vi "Modbus Initialization VI.vi"(8 "error in (no error)":errorcluster, 10 "Custom XML":string, 11 "Device Item Ref in":T1 format="%.0x") -> (0 "error out":errorcluster, 3 "Device Item Ref out":T1 format="%.0x")   [LabVIEW 2014, in "Modbus System Explorer.lvlib"]
uses:
  Modbus System Explorer.lvlib
  <vilib>/NI Veristand/Custom Device API/Custom Device Item Ref.ctl
  <vilib>/NI Veristand/Custom Device API/Custom Device Channel.ctl
  <vilib>/NI Veristand/Custom Device API/Custom Device Channel Type.ctl
  Glyphs/Modbus Property Names.vi
  Shared/Modbus GUID Lookup.vi
  <vilib>/NI Veristand/Custom Device API/Set Item Property (String).vi
  <vilib>/NI Veristand/Custom Device API/Set Item Property (Path).vi
  <vilib>/NI Veristand/Custom Device API/Custom Device API.lvlib
  Shared/Modbus Shared.lvlib
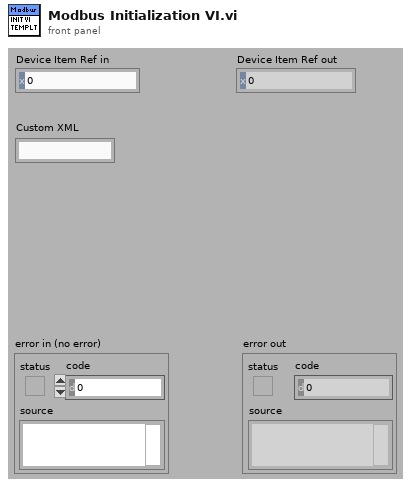
[diagram p1: front panel]
types:
  T1 = typedef "Custom Device API.lvlib/Custom Device Item Ref.ctl" = u64
  T2 = typedef "Custom Device API.lvlib/Custom Device Channel.ctl" = cluster{"Type":T3, "Units":string, "Default Value":dbl, "Faultable":bool, "Scalable":bool}
  T3 = typedef "Custom Device API.lvlib/Custom Device Channel Type.ctl" = enum16{"Input", "Output"}
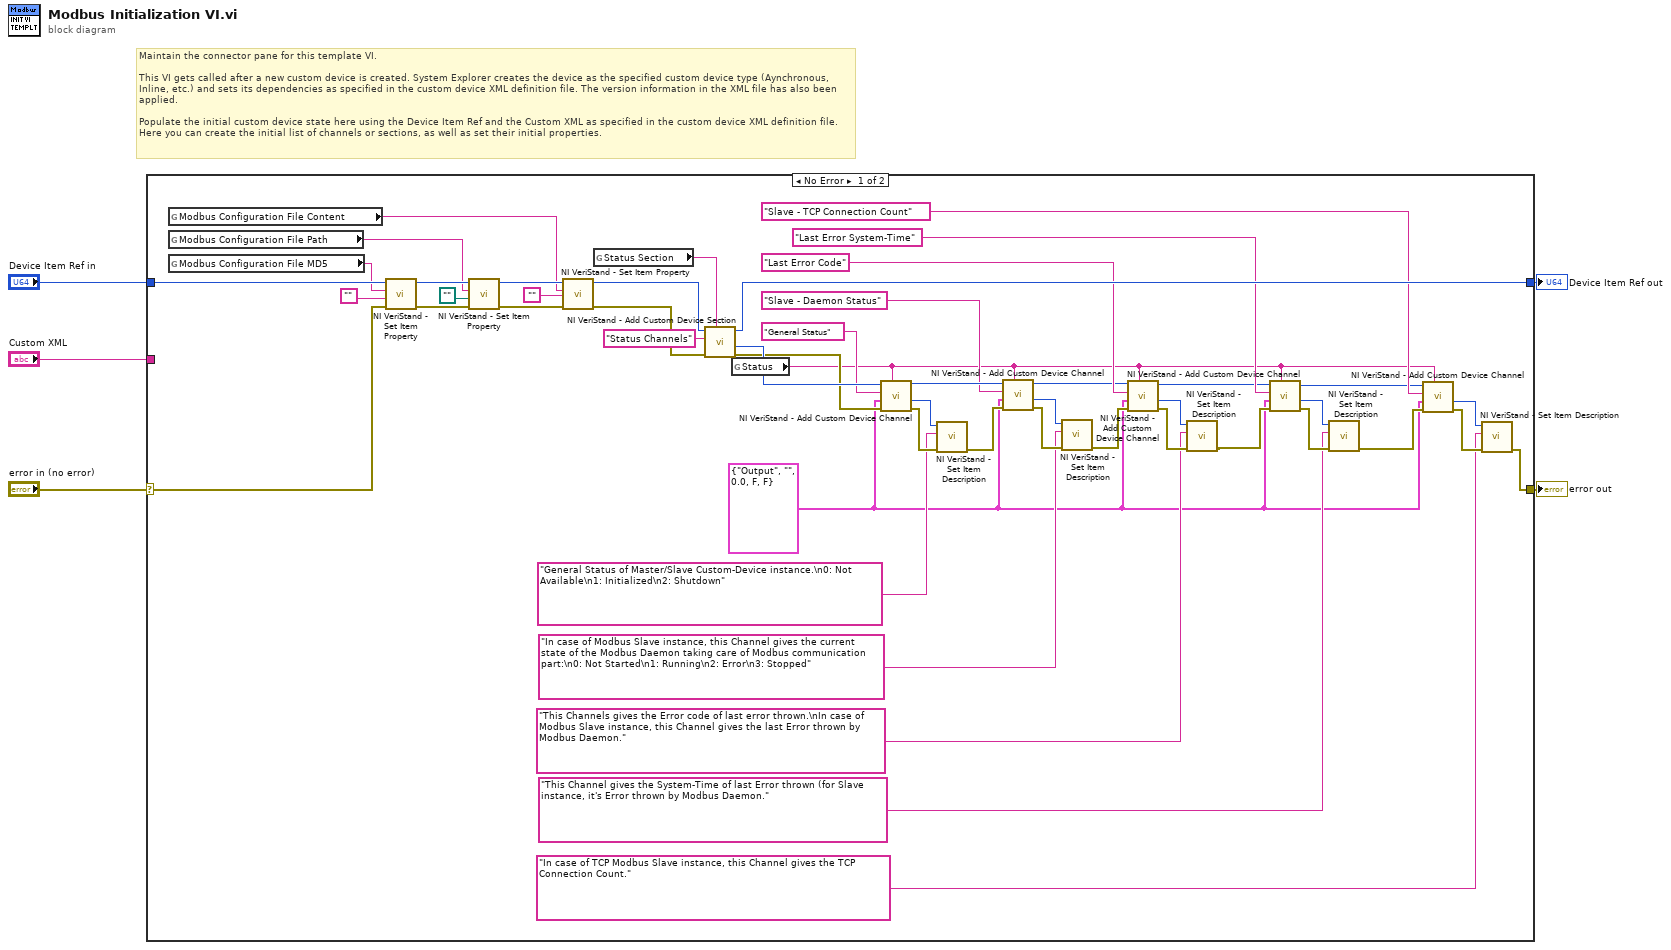
[diagram p0: block diagram]
diagram:
  # "Maintain the connector pane for this template VI.\n\nThis VI gets called after a new custom device is created. System Explorer creates the device as the specified custom device type (Aynchronous, Inline, etc.) and sets its dependencies as specified in the custom device XML definition file. The version information in the XML file has also been applied.\n\nPopulate the initial custom device state here using the Device Item Ref and the Custom XML as specified in the custom device XML definition file. Here you can create the initial list of channels or sections, as well as set their initial properties."
  n1 = case shown="No Error" "error in (no error)" {
    selector: "error in (no error)" -> [w52 w57]
    tunnel: [w9 w57] -> w5
    tunnel: [w41 w56] -> w3
    tunnel: "Device Item Ref in" -> [w55 w56]
    tunnel: "Custom XML" -> [_ _]
    frame No Error {
      w7 = T2 {"Type"=enum."Output", "Units"="", "Default Value"=0.0, "Faultable"=FALSE, "Scalable"=FALSE} ("Channel")
      n2 = global read "Modbus Property Names.vi" "Modbus Configuration File Content"() -> (w46:string)
      n3 = global read "Modbus Property Names.vi" "Modbus Configuration File Path"() -> (w49:string)
      n4 = global read "Modbus Property Names.vi" "Modbus Configuration File MD5"() -> (w54:string)
      n5 = call-poly <vilib>:"NI VeriStand - Set Item Property.vi"("error in (no error)"=w52, "Value"="", "Property Name"=w54, "Item Ref in"=w55) -> ("error out"=w51:errorcluster, "Item Ref out"=w50:T1)  [unwired: 5 in, 1 out]
      n6 = call-poly <vilib>:"NI VeriStand - Set Item Property.vi"("error in (no error)"=w51, "Value"=path "", "Property Name"=w49, "Item Ref in"=w50) -> ("error out"=w47:errorcluster, "Item Ref out"=w48:T1)  [unwired: 5 in, 1 out]
      n7 = call-poly <vilib>:"NI VeriStand - Set Item Property.vi"("error in (no error)"=w47, "Value"="", "Property Name"=w46, "Item Ref in"=w48) -> ("error out"=w42:errorcluster, "Item Ref out"=w43:T1)  [unwired: 5 in, 1 out]
      n8 = global read "Modbus GUID Lookup.vi" "Status Section"() -> (w37:string)
      n9 = call <vilib>:"NI VeriStand - Add Custom Device Section.vi"("GUID (Default Section)"=w37, "error in (no error)"=w42, "Section Name"="Status Channels", "Parent Ref in"=w43) -> ("error out"=w38:errorcluster, "Section Ptr"=w39:T1, "Parent Ref out"=w41:T1)  [unwired: 4 in, 1 out]
      n10 = global read "Modbus GUID Lookup.vi" "Status"() -> (w11:string)
      n11 = call <vilib>:"NI VeriStand - Add Custom Device Channel.vi"("GUID (Default Channel)"=w11, "error in (no error)"=w38, "Channel"=w7, "Channel Name"="General Status", "Parent Ref in"=w39) -> ("error out"=w34:errorcluster, "Channel Ref"=w35:T1, "Parent Ref out"=w31:T1)  [unwired: 3 in, 1 out]
      n12 = call <vilib>:"NI VeriStand - Set Item Description.vi"("error in (no error)"=w34, "Description"="General Status of Master/Slave Custom-Device instance.\n0: Not Available\n1: Initialized\n2: Shutdown", "Item Ref in"=w35) -> ("error out"=w32:errorcluster)  [unwired: 6 in, 2 out]
      n13 = call <vilib>:"NI VeriStand - Add Custom Device Channel.vi"("GUID (Default Channel)"=w11, "error in (no error)"=w32, "Channel"=w7, "Channel Name"="Slave - Daemon Status", "Parent Ref in"=w31) -> ("error out"=w30:errorcluster, "Channel Ref"=w29:T1, "Parent Ref out"=w23:T1)  [unwired: 3 in, 1 out]
      n14 = call <vilib>:"NI VeriStand - Set Item Description.vi"("error in (no error)"=w30, "Description"="In case of Modbus Slave instance, this Channel gives the current state of the Modbus Daemon taking care of Modbus communication part:\n0: Not Started\n1: Running\n2: Error\n3: Stopped", "Item Ref in"=w29) -> ("error out"=w22:errorcluster)  [unwired: 6 in, 2 out]
      n15 = call <vilib>:"NI VeriStand - Add Custom Device Channel.vi"("GUID (Default Channel)"=w11, "error in (no error)"=w22, "Channel"=w7, "Channel Name"="Last Error Code", "Parent Ref in"=w23) -> ("error out"=w24:errorcluster, "Channel Ref"=w25:T1, "Parent Ref out"=w16:T1)  [unwired: 3 in, 1 out]
      n16 = call <vilib>:"NI VeriStand - Set Item Description.vi"("error in (no error)"=w24, "Description"="This Channels gives the Error code of last error thrown.\nIn case of Modbus Slave instance, this Channel gives the last Error thrown by Modbus Daemon.", "Item Ref in"=w25) -> ("error out"=w17:errorcluster)  [unwired: 6 in, 2 out]
      n17 = call <vilib>:"NI VeriStand - Add Custom Device Channel.vi"("GUID (Default Channel)"=w11, "error in (no error)"=w17, "Channel"=w7, "Channel Name"="Last Error System-Time", "Parent Ref in"=w16) -> ("error out"=w20:errorcluster, "Channel Ref"=w19:T1, "Parent Ref out"=w8:T1)  [unwired: 3 in, 1 out]
      n18 = call <vilib>:"NI VeriStand - Set Item Description.vi"("error in (no error)"=w20, "Description"="This Channel gives the System-Time of last Error thrown (for Slave instance, it's Error thrown by Modbus Daemon.", "Item Ref in"=w19) -> ("error out"=w10:errorcluster)  [unwired: 6 in, 2 out]
      n19 = call <vilib>:"NI VeriStand - Add Custom Device Channel.vi"("GUID (Default Channel)"=w11, "error in (no error)"=w10, "Channel"=w7, "Channel Name"="Slave - TCP Connection Count", "Parent Ref in"=w8) -> ("error out"=w12:errorcluster, "Channel Ref"=w13:T1)  [unwired: 3 in, 2 out]
      n20 = call <vilib>:"NI VeriStand - Set Item Description.vi"("error in (no error)"=w12, "Description"="In case of TCP Modbus Slave instance, this Channel gives the TCP Connection Count.", "Item Ref in"=w13) -> ("error out"=w9:errorcluster)  [unwired: 6 in, 2 out]
    }
    frame Error {
    }
  }
  "error out" <- w5
  "Device Item Ref out" <- w3
